vi "Tipping Mechanism.vi"(10 "Un-Tip":bool, 11 "Tip":bool=TRUE) -> ()   [LabVIEW 2012]
uses:
  <vilib>/Rock Robotics/WPI/Solenoid/Deprecated/WPI_SolenoidSetBool.vi
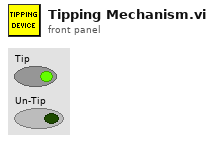
[diagram p1: front panel]
types:
  T1 = typedef "WPI_SolenoidDevRef.ctl" = cluster{"DevStatus":errorcluster, "Solenoid Module":T2, "Forward Solenoid Channel":T3, "Reverse Solenoid Channel":T3}
  T2 = typedef "FPGA_TypedefSolenoidModule.ctl" = enum16{"Solenoid Module 1", "Solenoid Module 2"}
  T3 = typedef "WPI_SolenoidChannel.ctl" = enum8{"Solenoid 1", "Solenoid 2", "Solenoid 3", "Solenoid 4", "Solenoid 5", "Solenoid 6", "Solenoid 7", "Solenoid 8", "Invalid"}
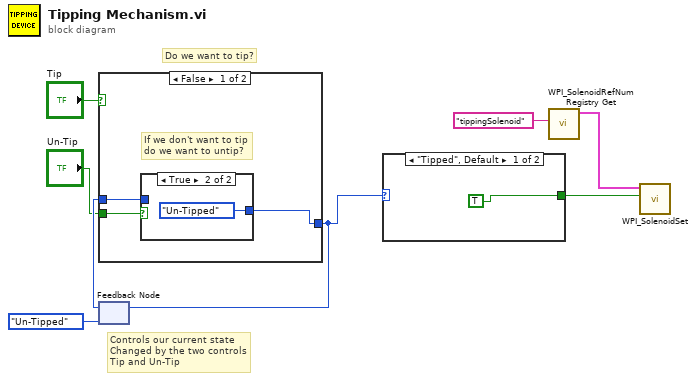
[diagram p0: block diagram]
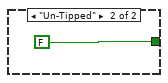
[diagram p2: hidden frame]
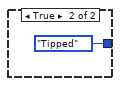
[diagram p4: hidden frame]
diagram:
  # "Do we want to tip?"
  # "Controls our current state\nChanged by the two controls\nTip and Un-Tip"
  n1 = feedback #1(enum16{"Tipped", "Un-Tipped"}."Un-Tipped") -> (w6:enum16{"Tipped", "Un-Tipped"})
  n2 = case shown="False" "Tip" {
    tunnel: w6 -> [w9 _]
    tunnel: [w10 enum16{"Tipped", "Un-Tipped"}."Tipped"] -> w2
    tunnel: "Un-Tip" -> [w11 _]
    frame False {
      # "If we don't want to tip\ndo we want to untip?"
      n3 = case shown="True" w11 {
        tunnel: [w12 enum16{"Tipped", "Un-Tipped"}."Un-Tipped"] -> w10
        tunnel: w9 -> [w12 _]
        frame False {
        }
        frame True {
        }
      }
    }
    frame True {
    }
  }
  n4 = feedback-in #1(w2) -> ()
  n5 = case shown="\"Tipped\", Default" w2 {
    tunnel: [TRUE FALSE] -> w1
    frame "Tipped", Default {
    }
    frame "Un-Tipped" {
    }
  }
  n6 = call <vilib>:"WPI_SolenoidRefNum Registry Get.vi"("refnum name"="tippingSolenoid") -> ("SolenoidDevRef"=w3:T1)  [unwired: 9 in, 1 out]
  n7 = call-poly <vilib>:"WPI_SolenoidSet.vi"("Value"=w1, "SolenoidDevRef"=w3) -> ()  [unwired: 8 in, 2 out]
